vi "ResizePicturetoPane.vi"(5 "Borders in Percent(T) or Pixels (F)":bool, 6 "Adjust":u16(ring) items=["Height", "Width", "Both"], 7 "Minimal":T1, 8 "error in (no error)":errorcluster, 9 "Borders":T2, 10 "Picture":refnum<vi>, 11 "PentaPanesGUI in":refnum<class "PentaPanes.lvclass">) -> (0 "error out":errorcluster, 3 "PentaPanesGUI out":refnum<class "PentaPanes.lvclass">)   [LabVIEW 2022 SP3, in "PentaPanesLibrary.lvlib" / "PentaPanes.lvclass"]
uses:
  PentaPanes.lvclass
  BordersCluster.ctl
  <vilib>/Utility/miscctls.llb/LVBoundsTypeDef.ctl
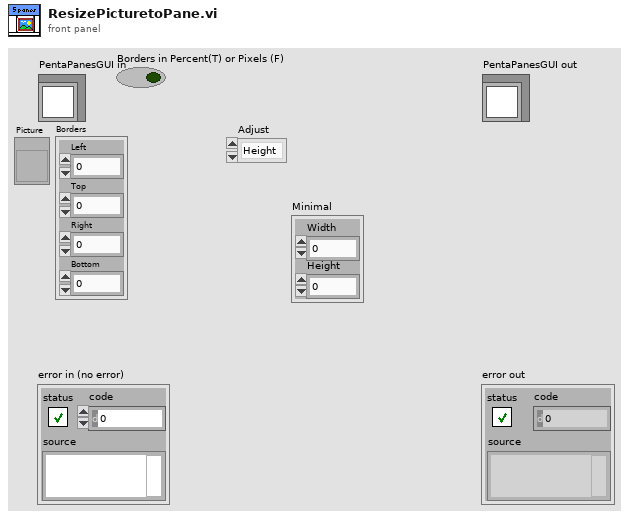
[diagram p1: front panel]
types:
  T1 = typedef "LVBoundsTypeDef.ctl" = cluster{"Width":i32, "Height":i32}
  T2 = typedef "PentaPanesLibrary.lvlib/PentaPanes.lvclass/BordersCluster.ctl" = cluster{"Left":i32, "Top":i32, "Right":i32, "Bottom":i32}
  T3 = typedef "LVBoundsTypeDef.ctl" = cluster{"Width":u32, "Height":u32}
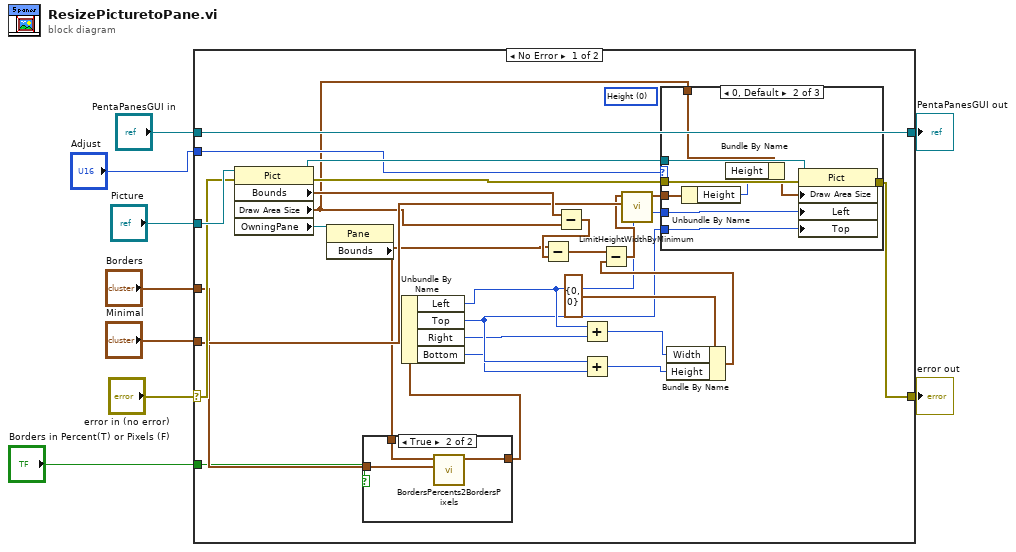
[diagram p0: block diagram]
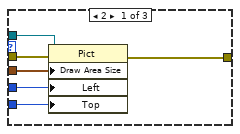
[diagram p3: hidden frame]
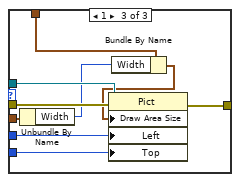
[diagram p4: hidden frame]
diagram:
  n1 = case shown="No Error" "error in (no error)" {
    selector: "error in (no error)" -> [w30 w66]
    tunnel: [w23 w66] -> w8
    tunnel: [w36 w65] -> w6
    tunnel: "PentaPanesGUI in" -> [w36 w65]
    tunnel: "Picture" -> [w31 _]
    tunnel: "Borders" -> [w13 _]
    tunnel: "Adjust" -> [w22 _]
    tunnel: "Minimal" -> [w20 _]
    tunnel: "Borders in Percent(T) or Pixels (F)" -> [w11 _]
    frame No Error {
      (unwired) u16 0 items=["Height", "Width", "Both"] ("Adjust")
      n2 = property class="Pict"(reference=w31, error in=w30) -> (reference out=w32:refnum<vi>, error out=w24:errorcluster, "Bounds"=w35:T3, "Draw Area Size"=w10:T3, "OwningPane"=w33:refnum<vi>)
      n3 = property class="Pane"(reference=w33) -> ("Bounds"=w16:T3)  [unwired: 1 in, 2 out]
      n4 = case shown="True" w11 {
        tunnel: w16 -> [_ w40]
        tunnel: w13 -> [w37 w39]
        tunnel: [w37 w38] -> w12
        frame False {
        }
        frame True {
          n5 = call "BordersPercents2BordersPixels.vi"("Borders in"=w39, "Bounds"=w40) -> ("Borders out"=w38:T2)  [unwired: 9 in]
        }
      }
      n6 = Unbundle By Name(w12) -> ("Left"=w18:i32, "Top"=w17:i32, "Right"=w15:i32, "Bottom"=w14:i32)
      n7 = Subtract(x=w35, y=w10) -> (x-y=w34:T3)
      n8 = Subtract(x=w16, y=w34) -> (x-y=w26:T3)
      n9 = Add(x=w18, y=w15) -> (x+y=w28:i32)
      n10 = Add(x=w17, y=w14) -> (x+y=w27:i32)
      n11 = Bundle By Name(cluster=T1 {"Width"=0, "Height"=0} ("x-y"), "Width"=w28, "Height"=w27) -> (w25:T1)
      n12 = Subtract(x=w26, y=w25) -> (x-y=w19:T3)
      n13 = call "LimitHeightWidthByMinimum.vi"("Minimal"=w20, "Height Width in"=w19) -> ("Limited Height Width out"=w21:T1)  [unwired: 9 in]
      n14 = case shown="0, Default" w22 {
        tunnel: w32 -> [w46 w55 w64]
        tunnel: w21 -> [w45 w50 w59]
        tunnel: w18 -> [w44 w54 w63]
        tunnel: w17 -> [w43 w53 w62]
        tunnel: w24 -> [w42 w52 w61]
        tunnel: [w41 w51 w60] -> w23
        tunnel: w10 -> [_ w48 w58]
        frame 2 {
          n15 = property class="Pict"(reference=w46, error in=w42, "Draw Area Size"=w45, "Left"=w44, "Top"=w43) -> (error out=w41:errorcluster)  [unwired: 1 out]
        }
        frame 0, Default {
          n16 = Unbundle By Name(w50) -> ("Height"=w47:i32)
          n17 = Bundle By Name(cluster=w48, "Height"=w47) -> (w49:T3)
          n18 = property class="Pict"(reference=w55, error in=w52, "Draw Area Size"=w49, "Left"=w54, "Top"=w53) -> (error out=w51:errorcluster)  [unwired: 1 out]
        }
        frame 1 {
          n19 = Unbundle By Name(w59) -> ("Width"=w57:i32)
          n20 = Bundle By Name(cluster=w58, "Width"=w57) -> (w56:T3)
          n21 = property class="Pict"(reference=w64, error in=w61, "Draw Area Size"=w56, "Left"=w63, "Top"=w62) -> (error out=w60:errorcluster)  [unwired: 1 out]
        }
      }
    }
    frame Error {
    }
  }
  "error out" <- w8
  "PentaPanesGUI out" <- w6
